vi "reverse4DImageChunk.vi"(11 "input":dbl[][][][](array[numeric])) -> (3 "output":dbl[][][][](array[numeric]))   [LabVIEW 2016]
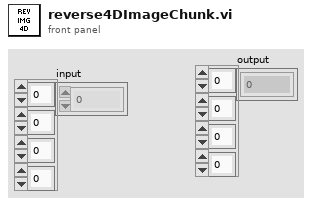
[diagram p1: front panel]
types:
  T1 = cluster{"[0]":i32, "[1]":i32, "[2]":i32, "[3]":i32}
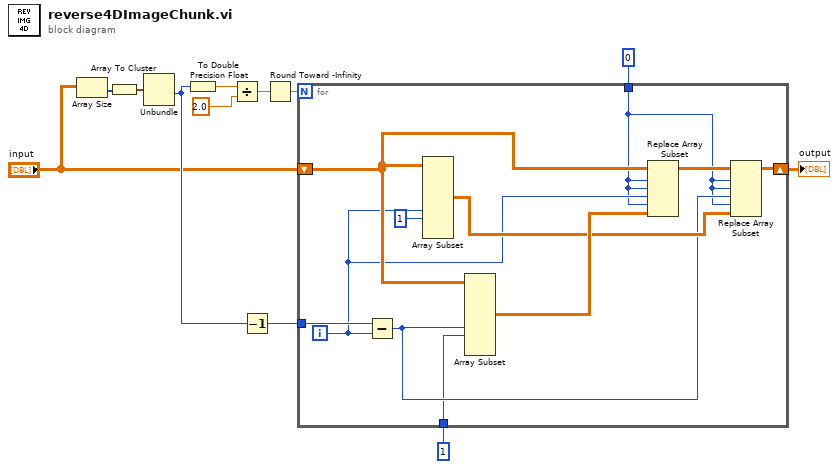
[diagram p0: block diagram]
diagram:
  n1 = Array Size(array="input") -> (size(s)=w10:i32[])
  n2 = Array To Cluster(array=w10) -> (cluster=w9:T1)
  n3 = Unbundle(w9) -> ("[2]"=w8:i32)  [unwired: 3 out]
  n4 = To Double Precision Float(number=w8) -> (double precision float=w3:dbl)
  n5 = Divide(x=w3, y=2.0) -> (x/y=w11:dbl)
  n6 = Decrement(x=w8) -> (x-1=w6:i32)
  n7 = Round Toward -Infinity(1:w11) -> (0:w12:dbl)
  n8 = for {
    N: w12 -> [_]
    shift-right: [w21] -> w7
    shift-left: "input" -> [w20]
    tunnel: w6 -> [w17]
    tunnel: 1 ("length") -> [w14]
    tunnel: 0 ("disabled index (vol)") -> [w13]
    i -> [w16]
    n9 = Subtract(x=w17, y=w16) -> (x-y=w15:i32)
    n10 = Array Subset(array=w20, index (dim 2)=w16, length (dim 2)=1 ("length")) -> (w18:dbl[][][][])  [unwired: 6 in]
    n11 = Array Subset(array=w20, index (dim 2)=w15, length (dim 2)=w14) -> (w19:dbl[][][][])  [unwired: 6 in]
    n12 = Replace Array Subset(array=w20, new element=w19, index (dim 0)=w13, index (dim 1)=w13, index (dim 2)=w16, index (dim 3)=w13) -> (w22:dbl[][][][])
    n13 = Replace Array Subset(array=w22, new element=w18, index (dim 0)=w13, index (dim 1)=w13, index (dim 2)=w15, index (dim 3)=w13) -> (w21:dbl[][][][])
  }
  "output" <- w7
